vi "GOOPUtil_GenericDestroy.vi"(0 "GOOPObject":refnum<class>, 5 "error in (no error)":errorcluster) -> (19 "error out":errorcluster)   [LabVIEW 2014, in "GOOPUtility.lvlib"]
doc: "When executed, the associated GOOP object Destroy method will be executed and the object will be deleted.\n\n\nThis is a collection of generic GOOP utility VIs. Please notice that it is important that the frontpanel of the Create, Destroy and GetObjectStatus is not removed when building an application."
uses:
  <vilib>/addons/GOOPUtility/GOOPUtility.lvlib
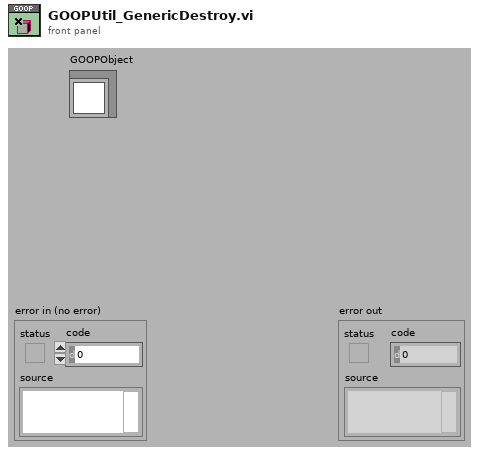
[diagram p1: front panel]
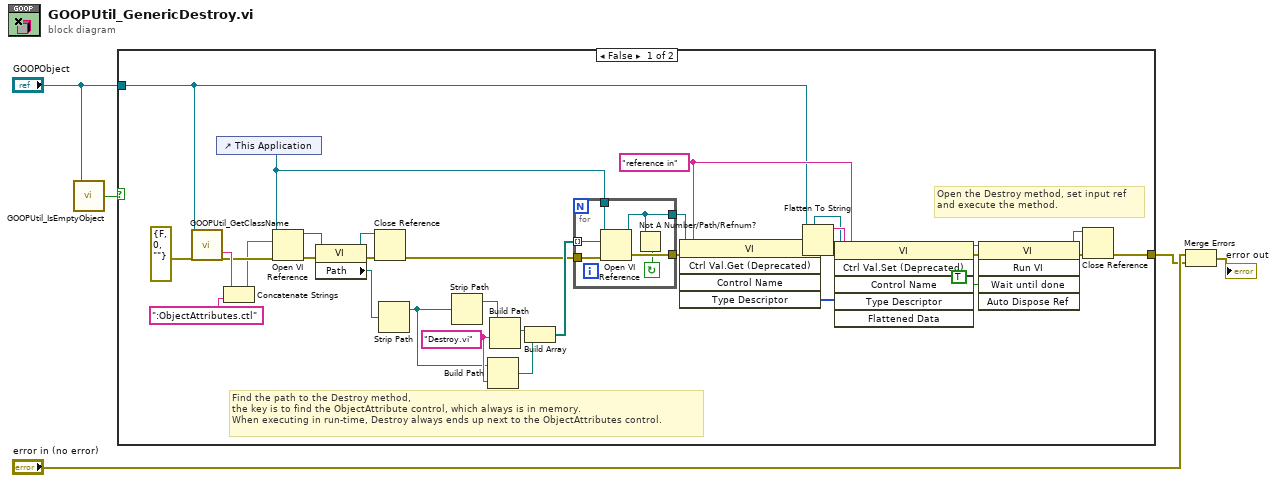
[diagram p0: block diagram]
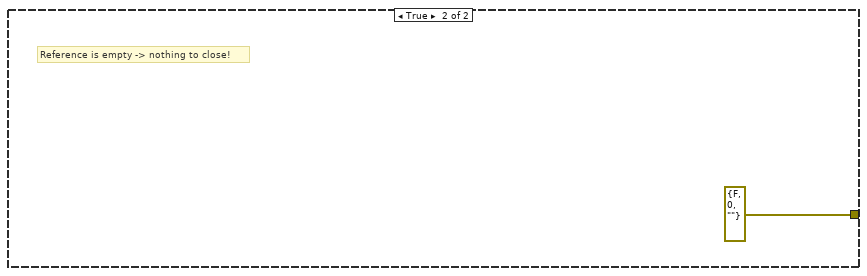
[diagram p2: hidden frame]
diagram:
  n1 = call <vilib>:"GOOPUtil_IsEmptyObject.vi"("LabVIEW Object"="GOOPObject") -> ("IsEmpty?"=w1:bool)
  n2 = case shown="False" w1 {
    tunnel: [w27 errorcluster {"status"=FALSE, "code"=0, "source"=""} ("error out")] -> w3
    tunnel: "GOOPObject" -> [w25 _]
    frame False {
      w14 = "Destroy.vi"
      w28 = "reference in" ("Control Name")
      # "Open the Destroy method, set input ref\nand execute the method."
      # "Find the path to the Destroy method,\nthe key is to find the ObjectAttribute control, which always is in memory.\nWhen executing in run-time, Destroy always ends up next to the ObjectAttributes control."
      n3 = call <vilib>:"GOOPUtil_GetClassName.vi"("LabVIEW Object"=w25, "error in (no error)"=errorcluster {"status"=FALSE, "code"=0, "source"=""}) -> ("Full Class Name"=w24:string, "error out"=w22:errorcluster)  [unwired: 13 in, 3 out]
      n4 = control-ref of="This Application"() -> (w9:refnum<vi>)
      n5 = Concatenate Strings(w24, ":ObjectAttributes.ctl" ("string")) -> (w21:string)
      n6 = Open VI Reference(application reference (local)=w9, vi path=w21, error in (no error)=w22) -> (vi reference=w19:refnum<vi>, error out=w20:errorcluster)  [unwired: 3 in]
      n7 = property class="VI"(reference=w19, error in=w20) -> (reference out=w17:refnum<vi>, error out=w18:errorcluster, "Path"=w7:path)
      n8 = Close Reference(reference=w17, error in (no error)=w18) -> (error out=w11:errorcluster)
      n9 = Strip Path(path=w7) -> (stripped path=w6:path)  [unwired: 1 out]
      n10 = Strip Path(path=w6) -> (stripped path=w13:path)  [unwired: 1 out]
      n11 = Build Path(base path=w6, name or relative path=w14) -> (appended path=w16:path)
      n12 = Build Path(base path=w13, name or relative path=w14) -> (appended path=w15:path)
      n13 = Build Array(w15, w16) -> (w12:path[])
      n14 = for {
        tunnel: w11 -> [w44]
        tunnel: [w43] -> w10
        tunnel: w9 -> [w42]
        tunnel: w12 -> [w41] mode=indexing
        tunnel: [w39] -> w8
        stop <- w40 continue-if-true
        n15 = Open VI Reference(application reference (local)=w42, vi path=w41, error in (no error)=w44) -> (vi reference=w39:refnum<vi>, error out=w43:errorcluster)  [unwired: 3 in]
        n16 = Not A Number/Path/Refnum?(number/path/refnum=w39) -> (NaN/Path/Refnum?=w40:bool)
      }
      n17 = invoke class="VI" method="Ctrl Val.Get (Deprecated)"(reference=w8, error in=w10, "Control Name"=w28) -> (reference out=w30:refnum<vi>, error out=w31:errorcluster, "Type Descriptor"=w29:i16[])  [unwired: 2 in, 2 out]
      n18 = Flatten To String(anything=w25, error in (no error)=w31) -> (data string=w32:string, error out=w33:errorcluster)  [unwired: 2 in, 1 out]
      n19 = invoke class="VI" method="Ctrl Val.Set (Deprecated)"(reference=w30, error in=w33, "Control Name"=w28, "Type Descriptor"=w29, "Flattened Data"=w32) -> (reference out=w36:refnum<vi>, error out=w37:errorcluster)  [unwired: 1 in, 4 out]
      n20 = invoke class="VI" method="Run VI"(reference=w36, error in=w37, "Wait until done"=TRUE ("Wait Until Done")) -> (reference out=w34:refnum<vi>, error out=w35:errorcluster)  [unwired: 2 in, 3 out]
      n21 = Close Reference(reference=w34, error in (no error)=w35) -> (error out=w27:errorcluster)
    }
    frame True {
      # "Reference is empty -> nothing to close!"
    }
  }
  n22 = Merge Errors("error in (no error)", w3) -> (→"error out":errorcluster)
